vi "Pneumatic Control.vi"(8 "error in":errorcluster, 10 "DIR":bool, 11 "ENA":bool) -> (0 "error out":errorcluster)   [LabVIEW 2019]
uses:
  KNRm_ReMi_OS6_436Motor.lvlibp/KNRm_ReMi_Toolkit/IO/LowLevel/IO_Channel_AO.ctl
  KNRm_ReMi_OS6_436Motor.lvlibp
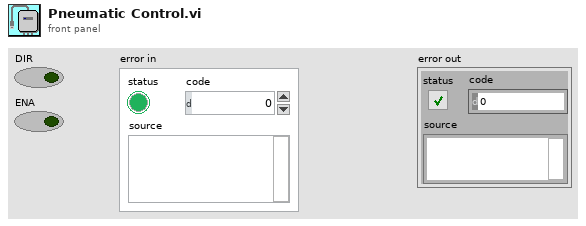
[diagram p1: front panel]
types:
  T1 = typedef "KNRm_ReMi_OS6_436Motor.lvlibp/IO_Channel_AO.ctl" = enum16{"AUX_AO_0", "AUX_AO_1", "AUX_AO_2", "AUX_AO_3"}
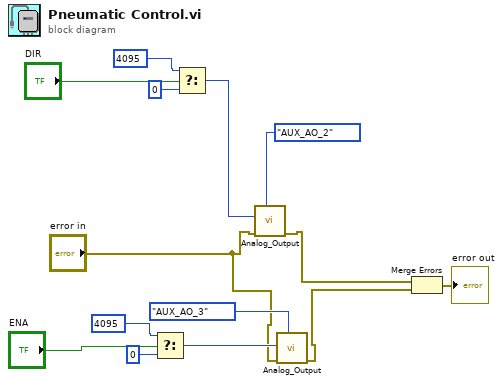
[diagram p0: block diagram]
diagram:
  n1 = Select(t=u16 4095 ("AO.VAL (1/819)V"), s="ENA", f=u16 0) -> (s? t:f=w6:u16)
  n2 = Select(t=u16 4095 ("AO.VAL (1/819)V"), s="DIR", f=u16 0) -> (s? t:f=w4:u16)
  n3 = call "Analog_Output.vi"("AO Channel"=IO_Channel_AO."AUX_AO_2", "error in"="error in", "AO.VAL (1/819)V"=w4) -> ("error out"=w2:errorcluster)  [unwired: 8 in]
  n4 = call "Analog_Output.vi"("AO Channel"=IO_Channel_AO."AUX_AO_3", "error in"="error in", "AO.VAL (1/819)V"=w6) -> ("error out"=w7:errorcluster)  [unwired: 8 in]
  n5 = Merge Errors(w2, w7) -> (→"error out":errorcluster)
